vi "Check String Validity.vi"(6 "String Name for Error":string, 9 "Max Characters":i32=-1, 10 "Valid String Specification":T1, 11 "String":string) -> (2 "string error":errorcluster, 3 "Valid":bool)   [LabVIEW 2015, in "NI_AWS_Core.lvlib" / "HTTP Request.lvclass"]
uses:
  HTTP Request.lvclass
  Valid String Specification.ctl
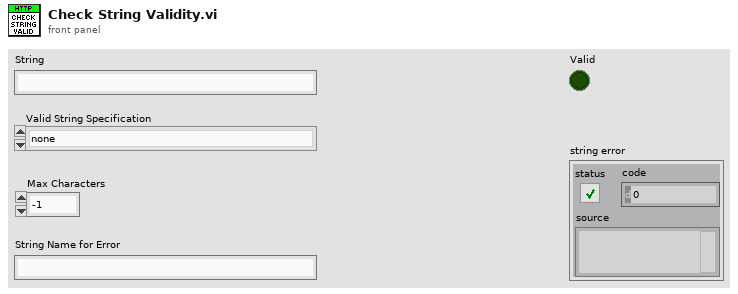
[diagram p1: front panel]
types:
  T1 = typedef "NI_AWS_Core.lvlib/HTTP Request.lvclass/Valid String Specification.ctl" = enum16{"none", "only [alphanumeric][-][_]", "only [alphanumeric][-][_][space]", "phone number +1xxxyyyzzzz"}
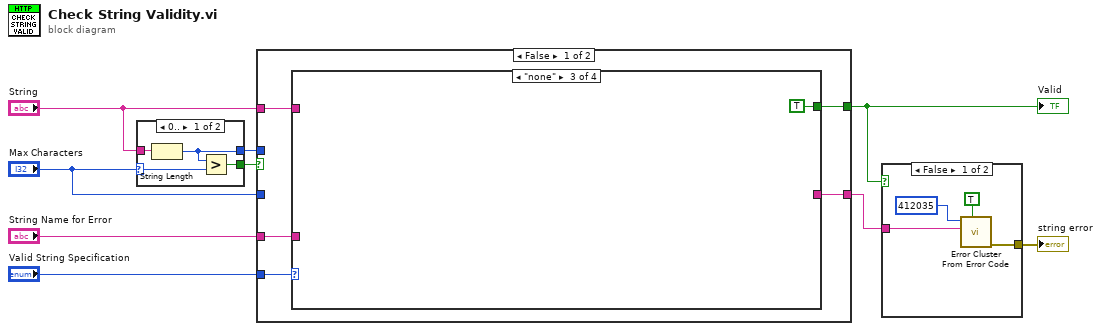
[diagram p0: block diagram]
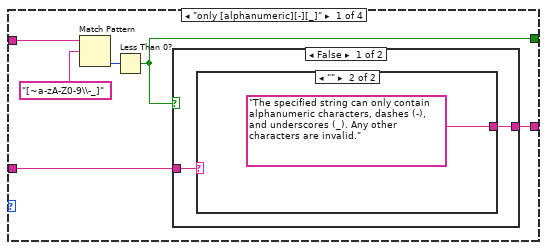
[diagram p4: hidden frame]
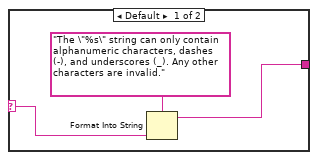
[diagram p5: hidden frame]
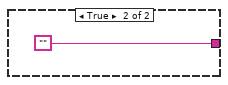
[diagram p6: hidden frame]
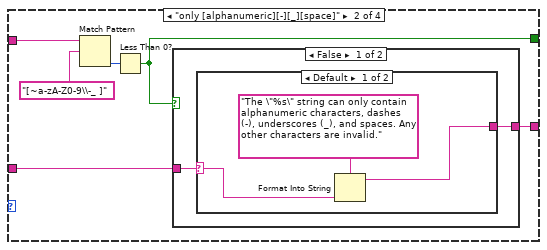
[diagram p7: hidden frame]
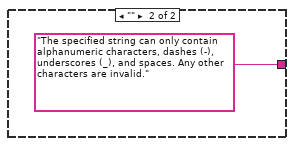
[diagram p8: hidden frame]
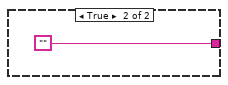
[diagram p9: hidden frame]
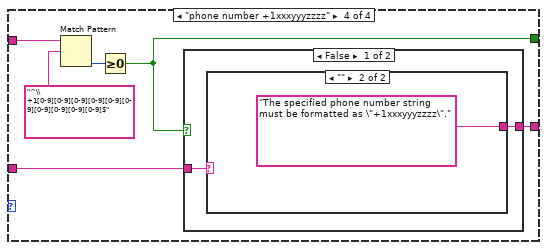
[diagram p10: hidden frame]
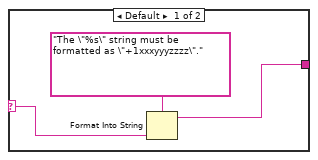
[diagram p11: hidden frame]
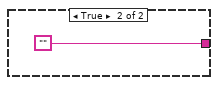
[diagram p12: hidden frame]
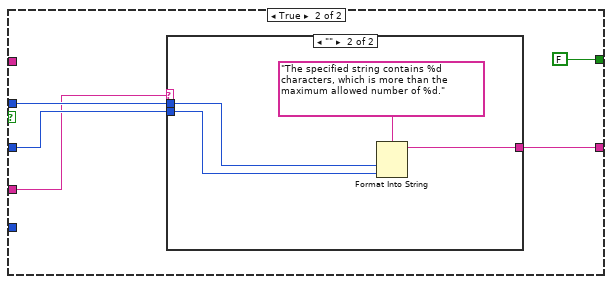
[diagram p13: hidden frame]
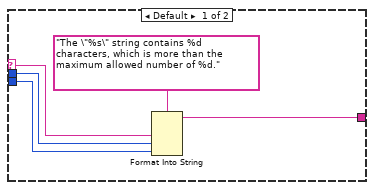
[diagram p14: hidden frame]
diagram:
  n1 = case shown="0.." "Max Characters" {
    selector: "Max Characters" -> [w11 _]
    tunnel: [w13 _] -> w9
    tunnel: "String" -> [w12 _]
    tunnel: [w10 _] -> w5
    frame 0.. {
      n2 = String Length(string=w12) -> (length=w10:i32)
      n3 = Greater?(x=w10, y=w11) -> (0:w13:bool)
    }
    frame ..-1 {
    }
  }
  n4 = case shown="False" w9 {
    tunnel: "String Name for Error" -> [w15 w60]
    tunnel: "String" -> [w17 _]
    tunnel: [w16 FALSE] -> w2
    tunnel: "Max Characters" -> [_ w61]
    tunnel: w5 -> [_ w62]
    tunnel: "Valid String Specification" -> [w18 _]
    tunnel: [w14 w59] -> w1
    frame False {
      n5 = case shown="\"none\"" w18 {
        tunnel: w17 -> [w24 w37 _ w49]
        tunnel: [w20 w33 TRUE w46] -> w16
        tunnel: w15 -> [w21 w34 _ w50]
        tunnel: [w19 w32 _ w51] -> w14
        frame "only [alphanumeric][-][_]" {
          n6 = Match Pattern(string=w24, regular expression="[~a-zA-Z0-9\\-_]") -> (offset past match=w22:i32)  [unwired: 1 in, 3 out]
          n7 = Less Than 0?(x=w22) -> (x < 0?=w20:bool)
          n8 = case shown="False" w20 {
            tunnel: w21 -> [w26 _]
            tunnel: [w25 ""] -> w19
            frame False {
              n9 = case shown="\"\"" w26 {
                selector: w26 -> [w28 _]
                tunnel: [w27 "The specified string can only contain alphanumeric characters, dashes (-), and underscores (_). Any other characters are invalid." ("error message (\"\")")] -> w25
                frame Default {
                  n10 = Format Into String(format string="The \"%s\" string can only contain alphanumeric characters, dashes (-), and underscores (_). Any other characters are invalid.", w28) -> (resulting string=w27:string)  [unwired: 2 in, 1 out]
                }
                frame "" {
                }
              }
            }
            frame True {
            }
          }
        }
        frame "only [alphanumeric][-][_][space]" {
          n11 = Match Pattern(string=w37, regular expression="[~a-zA-Z0-9\\-_ ]") -> (offset past match=w35:i32)  [unwired: 1 in, 3 out]
          n12 = Less Than 0?(x=w35) -> (x < 0?=w33:bool)
          n13 = case shown="False" w33 {
            tunnel: w34 -> [w39 _]
            tunnel: [w38 ""] -> w32
            frame False {
              n14 = case shown="Default" w39 {
                selector: w39 -> [w41 _]
                tunnel: [w40 "The specified string can only contain alphanumeric characters, dashes (-), underscores (_), and spaces. Any other characters are invalid." ("error message (\"\")")] -> w38
                frame Default {
                  n15 = Format Into String(format string="The \"%s\" string can only contain alphanumeric characters, dashes (-), underscores (_), and spaces. Any other characters are invalid.", w41) -> (resulting string=w40:string)  [unwired: 2 in, 1 out]
                }
                frame "" {
                }
              }
            }
            frame True {
            }
          }
        }
        frame "none" {
        }
        frame "phone number +1xxxyyyzzzz" {
          n16 = Match Pattern(string=w49, regular expression="^\\+1[0-9][0-9][0-9][0-9][0-9][0-9][0-9][0-9][0-9][0-9]$") -> (offset past match=w47:i32)  [unwired: 1 in, 3 out]
          n17 = Greater Or Equal To 0?(x=w47) -> (x >= 0?=w46:bool)
          n18 = case shown="False" w46 {
            tunnel: [w53 ""] -> w51
            tunnel: w50 -> [w52 _]
            frame False {
              n19 = case shown="\"\"" w52 {
                selector: w52 -> [w55 _]
                tunnel: [w54 "The specified phone number string must be formatted as \"+1xxxyyyzzzz\"." ("error message (\"\")")] -> w53
                frame Default {
                  n20 = Format Into String(format string="The \"%s\" string must be formatted as \"+1xxxyyyzzzz\".", w55) -> (resulting string=w54:string)  [unwired: 2 in, 1 out]
                }
                frame "" {
                }
              }
            }
            frame True {
            }
          }
        }
      }
    }
    frame True {
      n21 = case shown="\"\"" w60 {
        selector: w60 -> [w67 _]
        tunnel: w62 -> [w66 w69]
        tunnel: w61 -> [w65 w70]
        tunnel: [w64 w71] -> w59
        frame Default {
          n22 = Format Into String(format string="The \"%s\" string contains %d characters, which is more than the maximum allowed number of %d.", w67, w66, w65) -> (resulting string=w64:string)  [unwired: 2 in, 1 out]
        }
        frame "" {
          n23 = Format Into String(format string="The specified string contains %d characters, which is more than the maximum allowed number of %d.", w69, w70) -> (resulting string=w71:string)  [unwired: 2 in, 1 out]
        }
      }
    }
  }
  "Valid" <- w2
  n24 = case shown="False" w2 {
    tunnel: [w76 _] -> w3
    tunnel: w1 -> [w73 _]
    frame False {
      n25 = call <vilib>:"Error Cluster From Error Code.vi"("show call chain? (False)"=TRUE, "error message (\"\")"=w73, "error code (0)"=412035) -> ("error out"=w76:errorcluster)  [unwired: 6 in]
    }
    frame True {
    }
  }
  "string error" <- w3
